vi "Generate Self-Signed Certificates.vi"() -> ()   [LabVIEW 2013]
uses:
  certificate -- cluster.ctl
  certificate signature request (CA) -- cluster.ctl
  encryption key -- cluster.ctl
  initca -- cluster.ctl
  certificate signature request (Server) -- cluster.ctl
  <vilib>/Platform/browser.llb/Open URL in Default Browser (path).vi
  <userlib>/_OpenG.lib/file/file.llb/Build Path - Traditional__ogtk.vi
  <userlib>/_OpenG.lib/file/file.llb/File Exists - Scalar__ogtk.vi
  <userlib>/_OpenG.lib/file/file.llb/Convert File Extension (String)__ogtk.vi
panel:
  out "Selected Certificate":string
  in  "Certificates and Keys":i32(listbox)
  in  "Open Explorer":bool
  in  "Servers":cluster{"hosts":string[], "name":string}[](array[cluster])
  in  "Root Private Key":path
  in  "Root Certificate":path
  in  "Generate Server Certificates":bool
  in  "Generate Root Certificate":bool
  in  "Common Name":string="lvtls-ca.example"
  in  "Hosts":string[](array[string])=["lvtls-ca.example", "www.lvtls-ca.example"]
  # "1- ROOT (CERTIFICATE AUTHORITY)\nIf you have a root certificate and private key, import it to generate server certificate files.\nIf you don't have a root certificate, fill in the fields below and generate one."
  # "3- SERVERS\nList each server you want to create certificates for."
  # "2- GENERATE ROOT CERTIFICATE\nIf you don't have a root certificate, fill in the fields below and generate one."
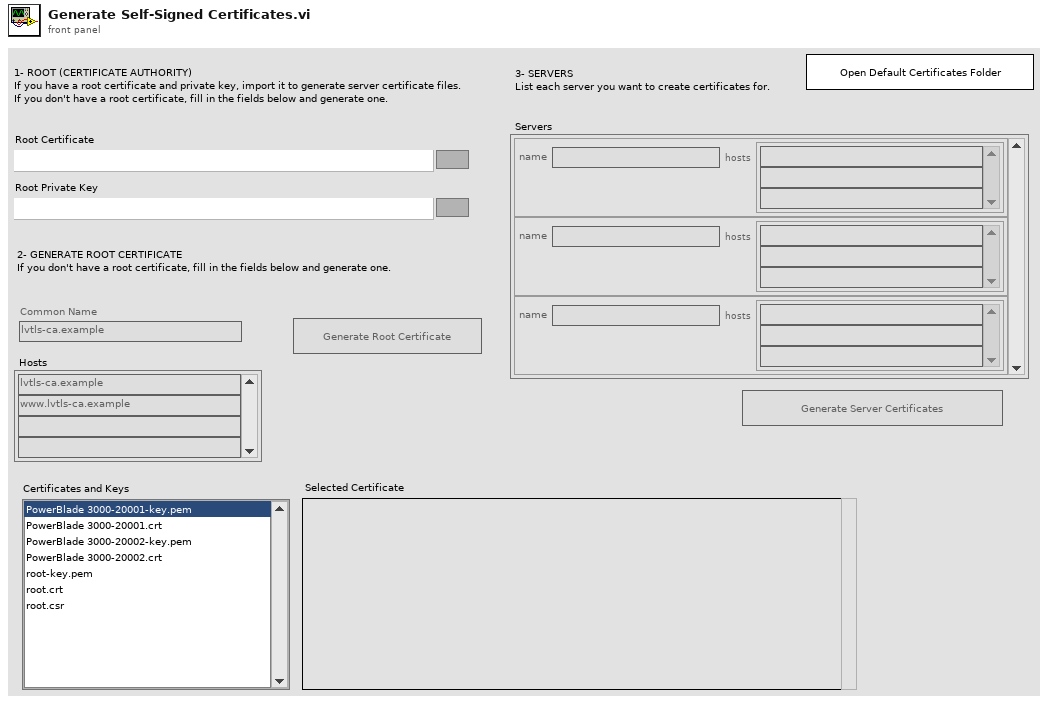
[diagram p1: front panel]
types:
  T1 = enum32{"Invalid", "Standard", "Closed", "Hidden", "Minimized", "Maximized"}
  T2 = enum32{"invalid app kind", "Development System", "Run Time System", "Student Edition", "Embedded LabVIEW", "Evaluation", "Custom"}
  T3 = enum16{"open", "replace", "create", "open or create", "replace or create", "replace or create with confirmation"}
  T4 = typedef "certificate signature request (CA) -- cluster.ctl" = cluster{"CN":string, "hosts":string[], "key":T5, "ca":T6}
  T5 = typedef "encryption key -- cluster.ctl" = cluster{"algo":string, "size":u32}
  T6 = typedef "initca -- cluster.ctl" = cluster{"pathlen":u8, "expiry":string}
  T7 = typedef "certificate signature request (Server) -- cluster.ctl" = cluster{"CN":string, "hosts":string[], "key":T5}
  T8 = typedef "certificate -- cluster.ctl" = cluster{"cert":string, "csr":string, "key":string}
  T9 = cluster{"Core":cluster{"Current VI Reference":refnum<vi>, "Close Panel on Exit?":bool}, "CA":T8, "Server":T8, "cfssl path":path, "temp folder":path, "Certificates Folder":path, "Root name":string, "Root Certificate":path, "Root Private Key":path, "Active CN":string, "Active Hosts":string[], "next":i32, "Processing Queue":cluster{"hosts":string[], "name":string}[]}
  T10 = cluster{"Current VI Reference":refnum<vi>, "Close Panel on Exit?":bool}
  T11 = enum8{"Enabled", "Disabled", "Disabled and Grayed Out"}
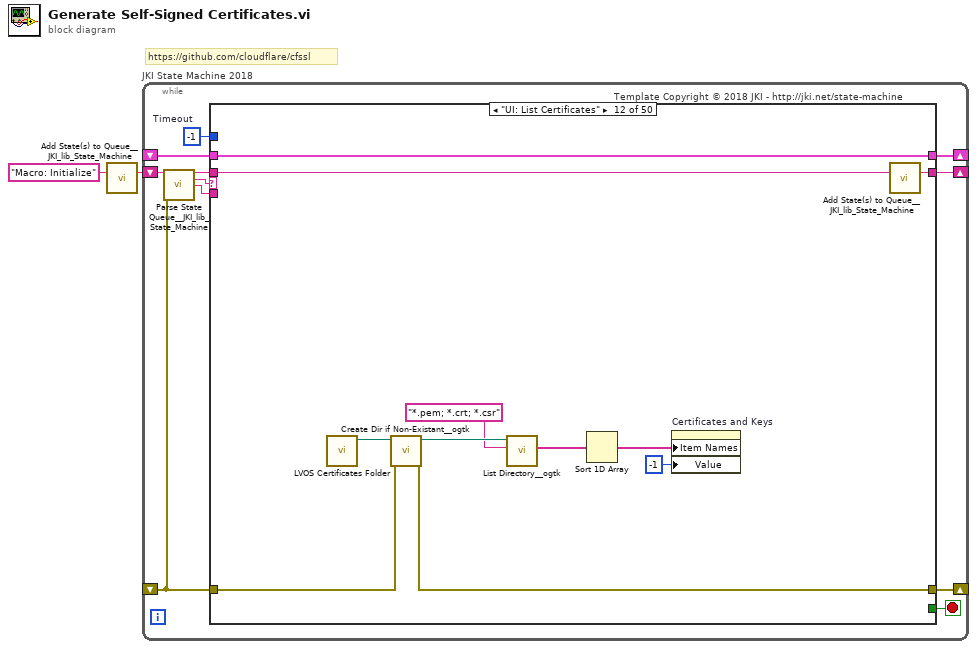
[diagram p0: block diagram]
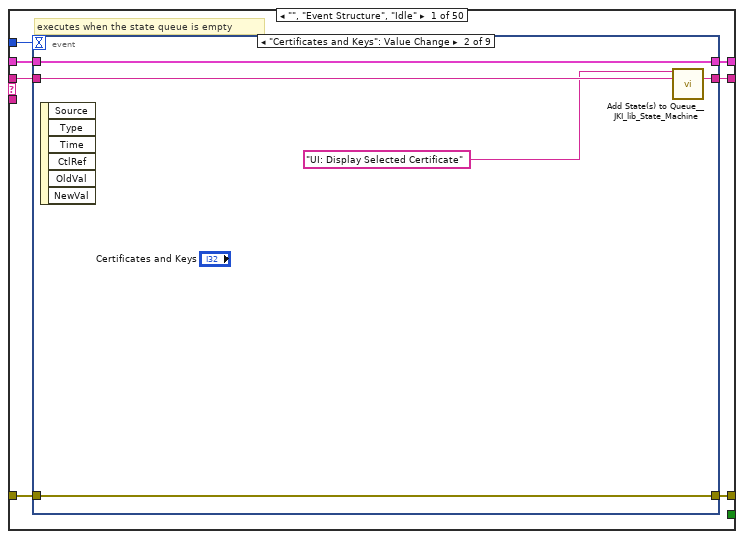
[diagram p2: hidden frame]
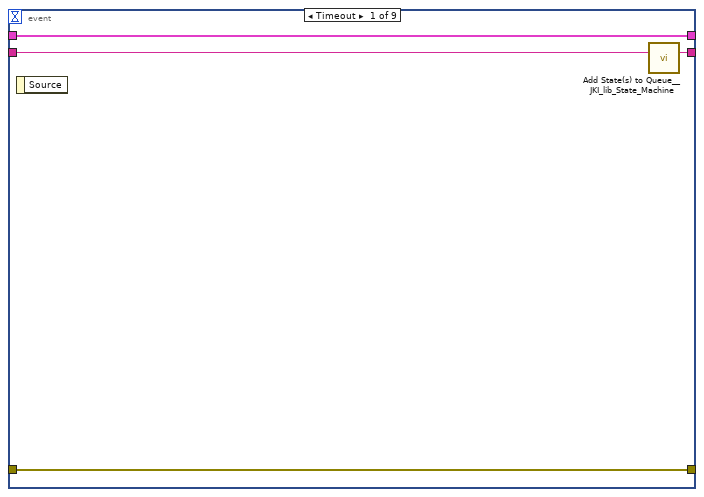
[diagram p3: hidden frame]
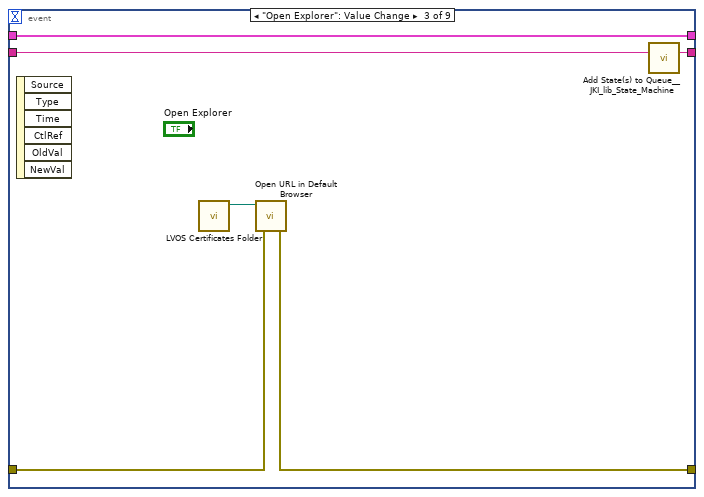
[diagram p4: hidden frame]
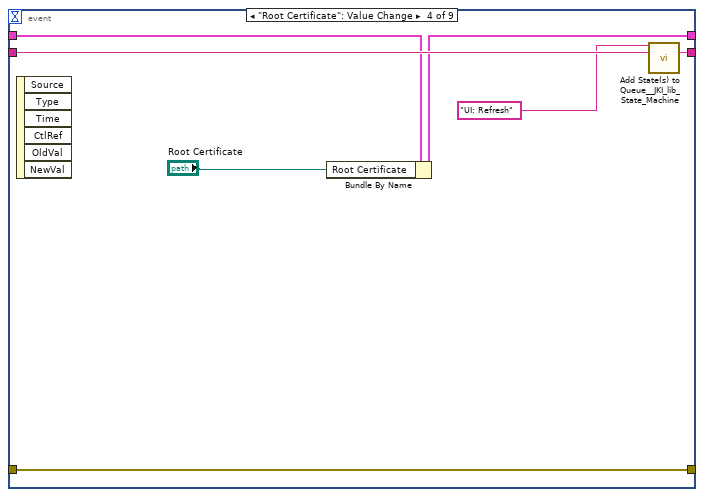
[diagram p5: hidden frame]
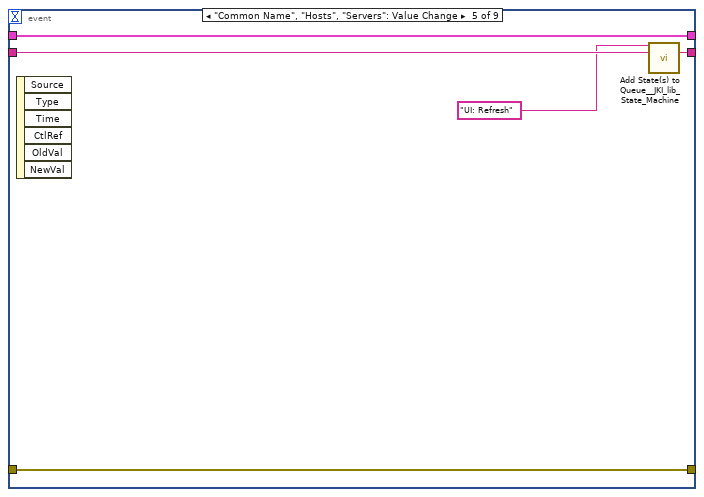
[diagram p6: hidden frame]
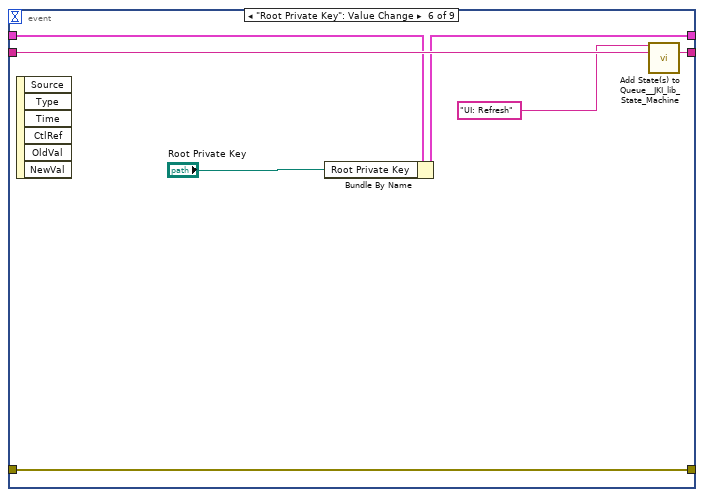
[diagram p7: hidden frame]
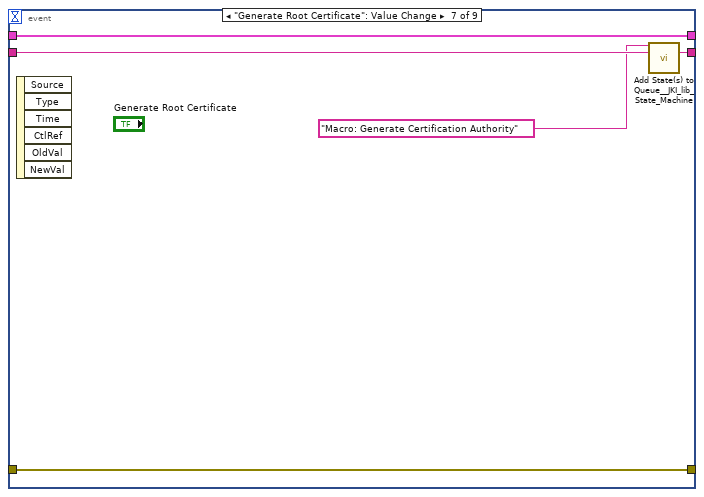
[diagram p8: hidden frame]
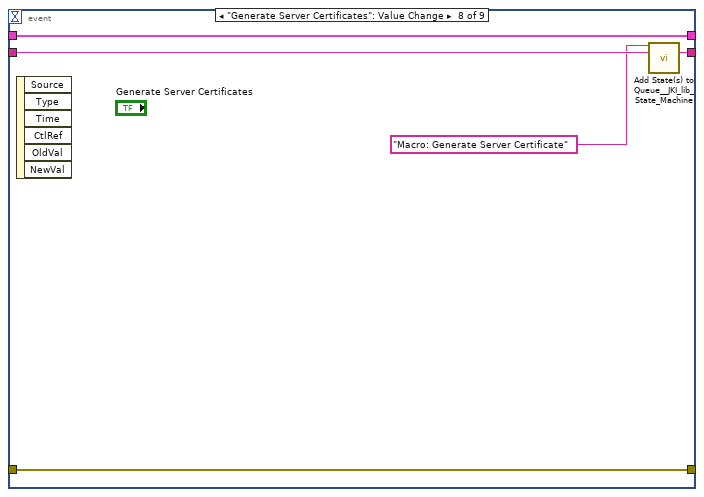
[diagram p9: hidden frame]
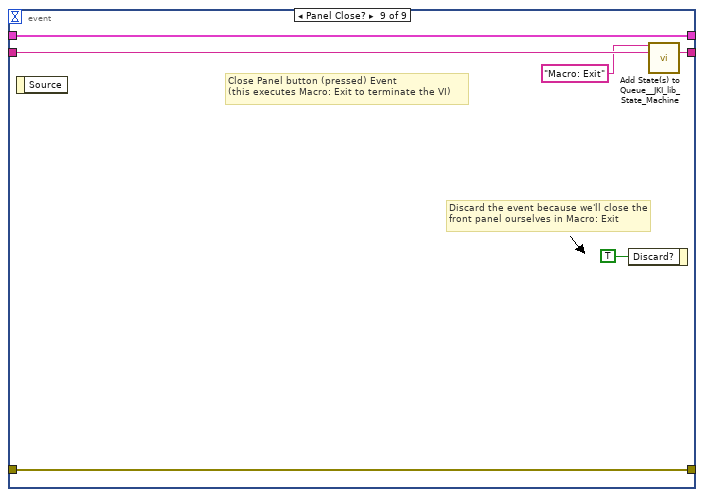
[diagram p10: hidden frame]
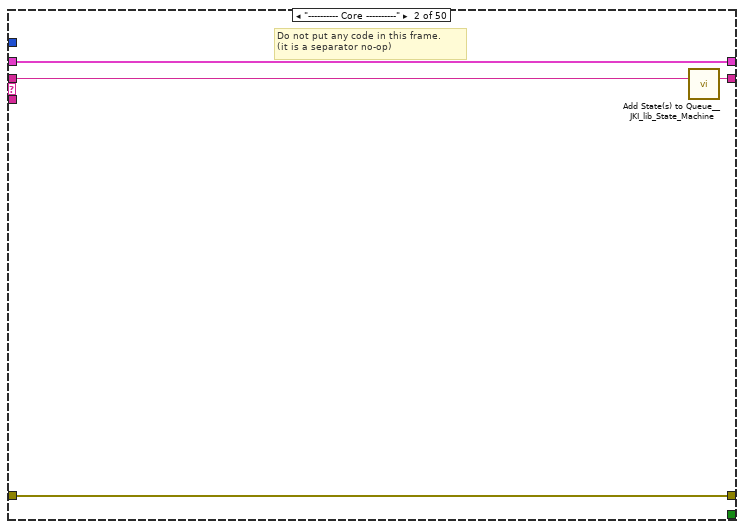
[diagram p11: hidden frame]
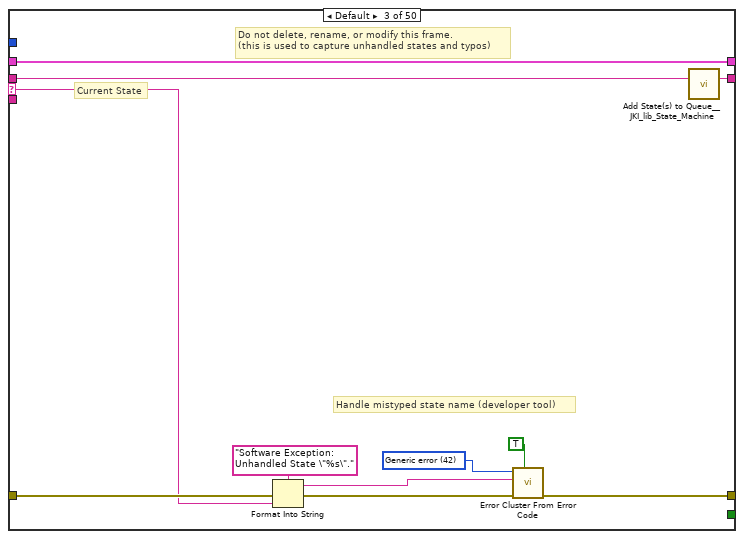
[diagram p12: hidden frame]
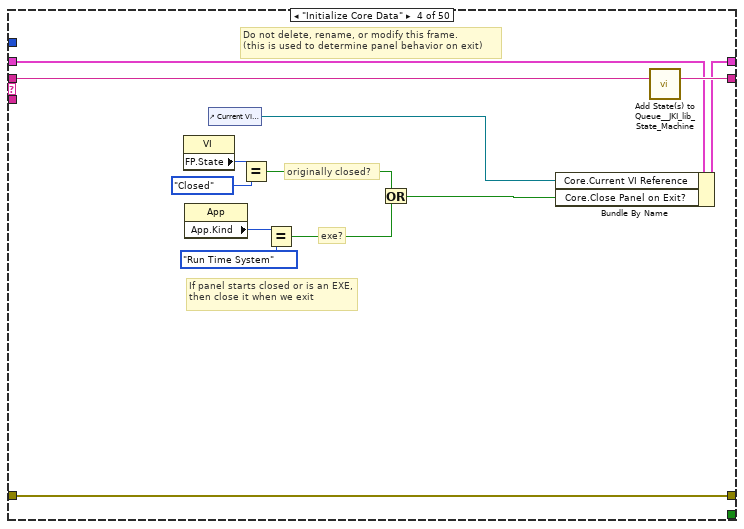
[diagram p13: hidden frame]
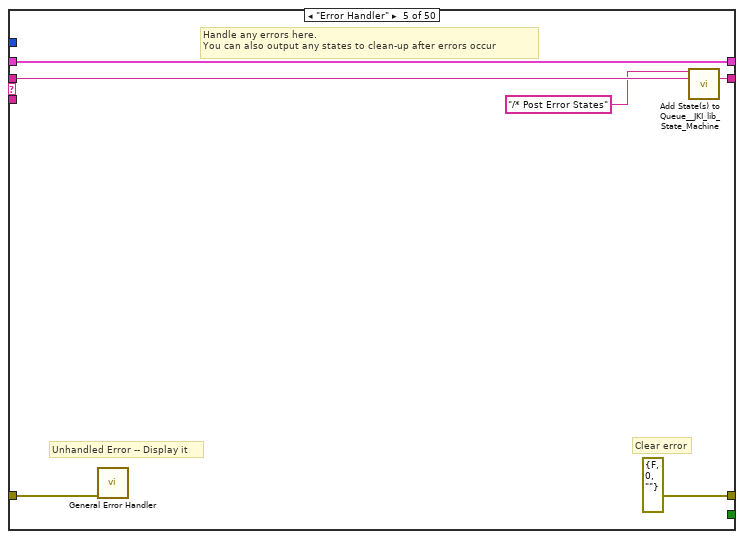
[diagram p14: hidden frame]
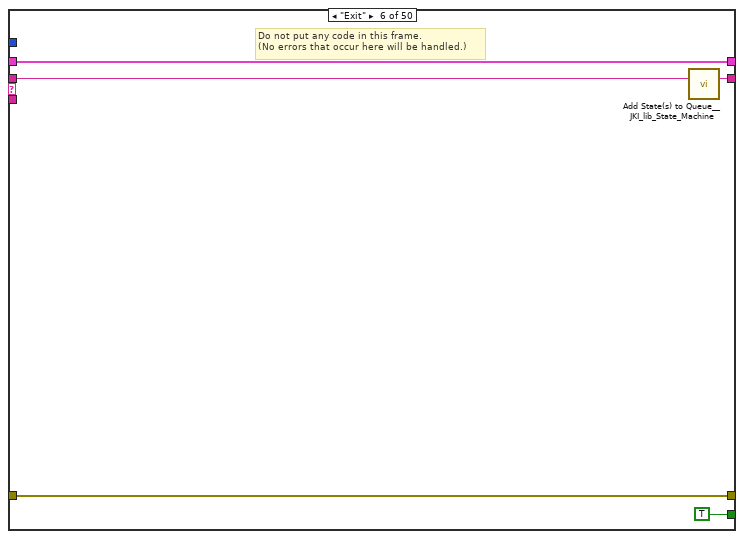
[diagram p15: hidden frame]
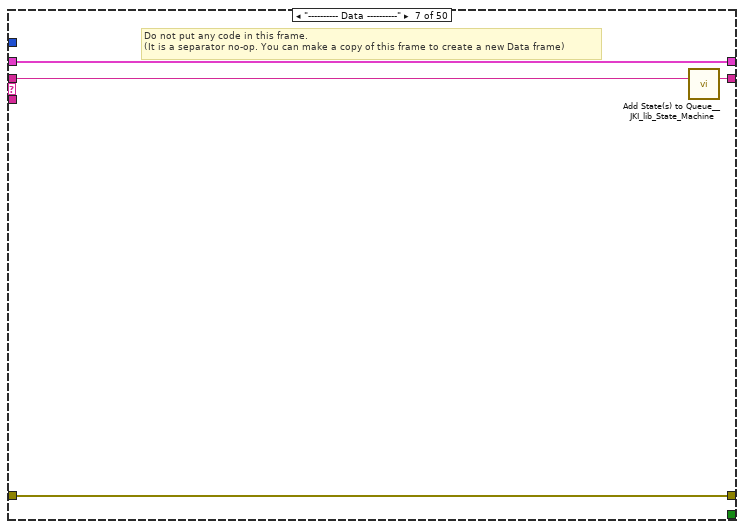
[diagram p16: hidden frame]
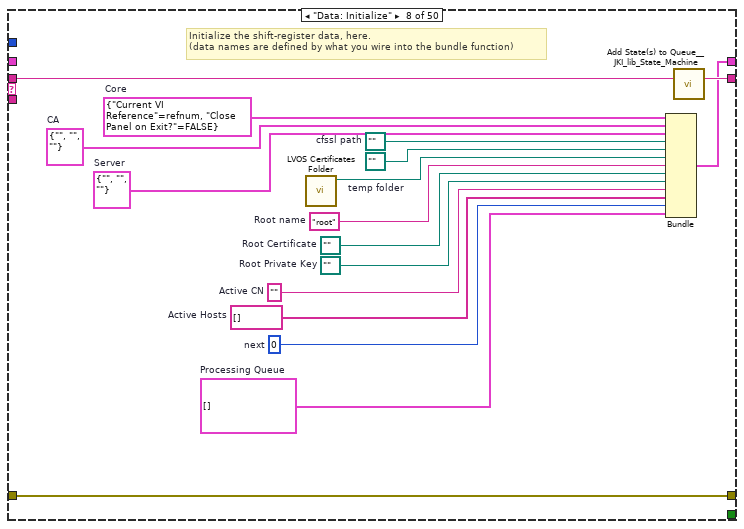
[diagram p17: hidden frame]
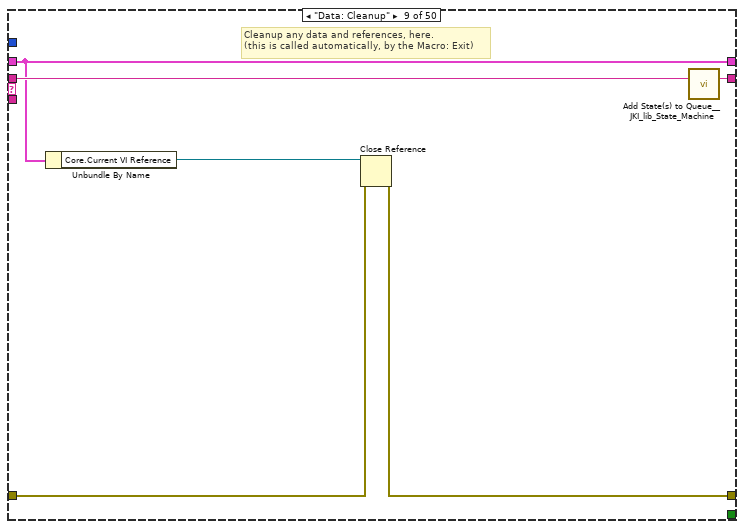
[diagram p18: hidden frame]
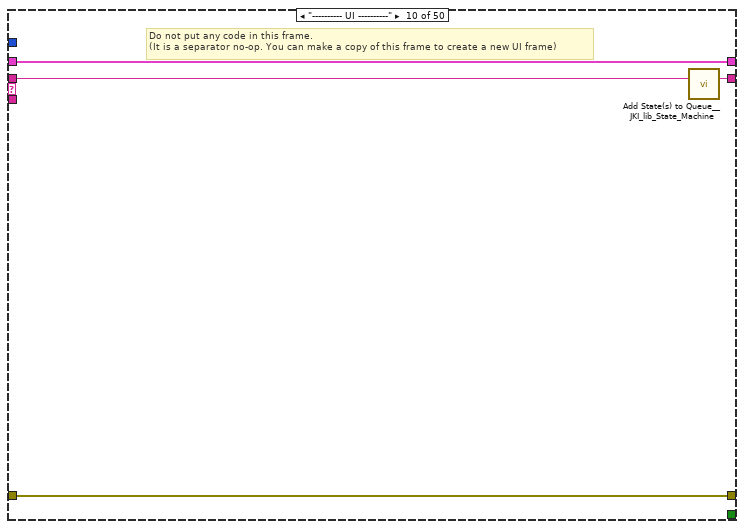
[diagram p19: hidden frame]
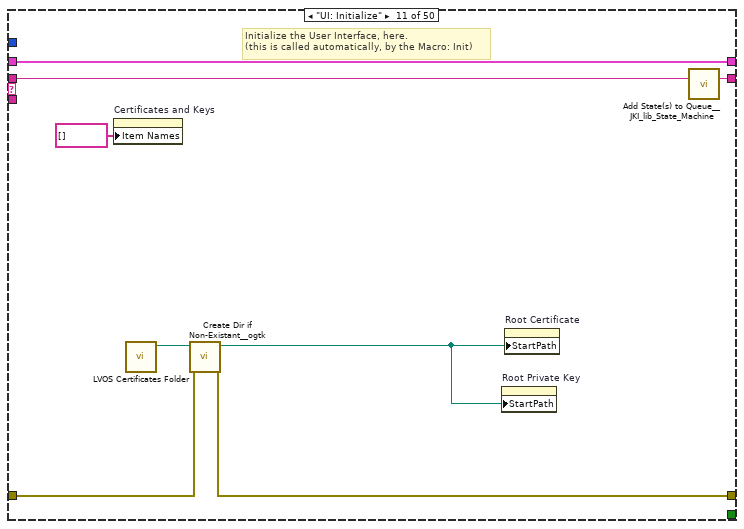
[diagram p20: hidden frame]
diagram:
  # "https://github.com/cloudflare/cfssl"
  n1 = call <vilib>:"Add State(s) to Queue__JKI_lib_State_Machine.vi"("State(s) in (\"\")"="Macro: Initialize") -> ("States Out"=w2:string)  [unwired: 14 in]
  n2 = while "JKI State Machine 2018" {
    shift-right: [w6] -> _
    shift-left: _ -> [w5]
    shift-right: [w9] -> _
    shift-left: _ -> [w3]
    shift-right: [w8] -> _
    shift-left: w2 -> [w10]
    stop <- w7 stop-if-true
    w4 = -1  # Timeout
    # "Template Copyright © 2018 JKI - http://jki.net/state-machine"
    n3 = call <vilib>:"Parse State Queue__JKI_lib_State_Machine.vi"("State Queue"=w10, "Error In (no error)"=w3) -> ("Remaining States"=w12:string, "Current State"=w13:string, "Arguments"=w11:string)  [unwired: 11 in]
    n4 = case shown="\"UI: List Certificates\"" w13 {
      selector: w13 -> [_ _ w75 _ _ _ _ _ _ _ _ _ _ _ _ _ _ _ _ _ _ _ _ _ _ _ _ _ _ _ _ _ _ _ _ _ _ _ _ _ _ _ _ _ _ _ _ _ _ _]
      tunnel: w12 -> [w20 w74 w79 w98 w104 w109 w113 w130 w136 w140 w148 w159 w167 w217 w221 w225 w230 w236 w247 w316 w321 w326 w334 w339 w348 w353 w364 w368 w376 w385 w395 w422 w437 w452 w475 w496 w513 w523 w537 w568 w591 w617 w640 w672 w689 w706 w723 w740 w757 w774]
      tunnel: w11 -> [_ _ _ _ _ _ _ _ _ _ _ _ _ _ _ _ _ w231 w241 _ _ _ _ _ _ _ _ _ _ _ _ _ _ _ _ _ _ _ _ _ _ _ _ _ _ _ _ _ _ _]
      tunnel: w5 -> [w18 w71 w77 w91 w101 w107 w110 _ w131 w137 w146 w157 w165 w206 w218 w222 w227 w234 w243 w313 w318 w323 w330 w336 w345 w350 w361 w365 w373 w383 w393 w418 w426 w442 w473 w494 w506 w518 w535 w538 w584 w613 w630 w655 w681 w698 w715 w732 w749 w766]
      tunnel: [w17 w72 w81 w95 errorcluster {"status"=FALSE, "code"=0, "source"=""} ("error out") w106 w111 w127 w132 w138 w142 w154 w162 w215 w219 w223 w228 w232 w244 w314 w319 w324 w332 w337 w346 w351 w362 w366 w374 w378 w389 w420 w423 w439 w453 w482 w499 w514 w526 w541 w586 w614 w619 w656 w676 w693 w710 w727 w744 w761] -> w9
      tunnel: w3 -> [w16 w72 w80 w95 w100 w106 w111 w127 w133 w138 w143 w155 w162 w215 w219 w223 w228 w233 w245 w314 w319 w324 w332 w337 w346 w351 w362 w366 w374 w379 w388 w420 w424 w440 w454 w483 w500 w514 w524 w545 w587 w615 w622 w659 w678 w695 w712 w729 w746 w763]
      tunnel: [w19 w73 w78 w97 w103 w108 w112 w129 w135 w139 w147 w158 w166 w216 w220 w224 w229 w235 w246 w315 w320 w325 w333 w338 w347 w352 w363 w367 w375 w384 w394 w421 w436 w451 w474 w495 w512 w522 w536 w567 w590 w616 w639 w671 w688 w705 w722 w739 w756 w773] -> w8
      tunnel: [_ _ _ _ _ TRUE _ _ _ _ _ _ _ _ _ _ _ _ _ _ _ _ _ _ _ _ _ _ _ _ _ _ _ _ _ _ _ _ _ _ _ _ _ _ _ _ _ _ _ _] -> w7
      tunnel: [w15 w71 w77 w96 w101 w107 w110 w128 w131 w137 w146 w157 w165 w206 w218 w222 w227 w234 w243 w313 w318 w323 w329 w336 w345 w350 w361 w365 w372 w382 w393 w419 w427 w443 w473 w494 w506 w521 w535 w538 w583 w612 w630 w655 w681 w698 w715 w732 w749 w766] -> w6
      tunnel: w4 -> [w14 _ _ _ _ _ _ _ _ _ _ _ _ _ _ _ _ _ _ _ _ _ _ _ _ _ _ _ _ _ _ _ _ _ _ _ _ _ _ _ _ _ _ _ _ _ _ _ _ _]
      frame "", "Event Structure", "Idle" {
        # "executes when the state queue is empty"
        n5 = event shown="[1] \"Certificates and Keys\": Value Change" {
          selector: _ -> [_ _ _ _ _ _ _ _ _]
          dyn-events: _ -> [_ _ _ _ _ _ _ _ _]
          timeout: w14 -> [_ _ _ _ _ _ _ _ _]
          tunnel: w20 -> [w24 w29 w35 w42 w47 w54 w59 w64 w70]
          tunnel: [w23 w28 w34 w41 w46 w53 w58 w63 w69] -> w19
          tunnel: w18 -> [w21 w26 w33 w39 w43 w51 w56 w61 w67]
          tunnel: [w22 w27 w30 w40 w45 w52 w57 w62 w68] -> w17
          tunnel: w16 -> [w22 w27 w31 w40 w45 w52 w57 w62 w68]
          tunnel: [w21 w26 w33 w38 w43 w50 w56 w61 w67] -> w15
          event Timeout {
            n6 = event-data() -> ()  [unwired: 1 in, 1 out]
            n7 = call <vilib>:"Add State(s) to Queue__JKI_lib_State_Machine.vi"("State(s) in (\"\")"=w24) -> ("States Out"=w23:string)  [unwired: 14 in]
          }
          event "Certificates and Keys": Value Change {
            n8 = event-data() -> ()  [unwired: 1 in, 6 out]
            n9 = call <vilib>:"Add State(s) to Queue__JKI_lib_State_Machine.vi"("State(s) in Front (\"\")"="UI: Display Selected Certificate", "State(s) in (\"\")"=w29) -> ("States Out"=w28:string)  [unwired: 13 in]
          }
          event "Open Explorer": Value Change {
            n10 = event-data() -> ()  [unwired: 1 in, 6 out]
            n11 = call "LVOS Certificates Folder.vi"() -> ("Certificates Folder"=w32:path)  [unwired: 11 in]
            n12 = call-poly <vilib>:"Open URL in Default Browser.vi"("error in (no error)"=w31, "path"=w32) -> ("error out"=w30:errorcluster)  [unwired: 4 in, 1 out]
            n13 = call <vilib>:"Add State(s) to Queue__JKI_lib_State_Machine.vi"("State(s) in (\"\")"=w35) -> ("States Out"=w34:string)  [unwired: 14 in]
          }
          event "Root Certificate": Value Change {
            n14 = event-data() -> ()  [unwired: 1 in, 6 out]
            n15 = Bundle By Name(cluster=w39, "Root Certificate"="Root Certificate") -> (w38:T9)
            n16 = call <vilib>:"Add State(s) to Queue__JKI_lib_State_Machine.vi"("State(s) in Front (\"\")"="UI: Refresh", "State(s) in (\"\")"=w42) -> ("States Out"=w41:string)  [unwired: 13 in]
          }
          event "Common Name", "Hosts", "Servers": Value Change {
            n17 = event-data() -> ()  [unwired: 1 in, 6 out]
            n18 = call <vilib>:"Add State(s) to Queue__JKI_lib_State_Machine.vi"("State(s) in Front (\"\")"="UI: Refresh", "State(s) in (\"\")"=w47) -> ("States Out"=w46:string)  [unwired: 13 in]
          }
          event "Root Private Key": Value Change {
            n19 = event-data() -> ()  [unwired: 1 in, 6 out]
            n20 = Bundle By Name(cluster=w51, "Root Private Key"="Root Private Key") -> (w50:T9)
            n21 = call <vilib>:"Add State(s) to Queue__JKI_lib_State_Machine.vi"("State(s) in Front (\"\")"="UI: Refresh", "State(s) in (\"\")"=w54) -> ("States Out"=w53:string)  [unwired: 13 in]
          }
          event "Generate Root Certificate": Value Change {
            n22 = event-data() -> ()  [unwired: 1 in, 6 out]
            n23 = call <vilib>:"Add State(s) to Queue__JKI_lib_State_Machine.vi"("State(s) in Front (\"\")"="Macro: Generate Certification Authority", "State(s) in (\"\")"=w59) -> ("States Out"=w58:string)  [unwired: 13 in]
          }
          event "Generate Server Certificates": Value Change {
            n24 = event-data() -> ()  [unwired: 1 in, 6 out]
            n25 = call <vilib>:"Add State(s) to Queue__JKI_lib_State_Machine.vi"("State(s) in Front (\"\")"="Macro: Generate Server Certificate", "State(s) in (\"\")"=w64) -> ("States Out"=w63:string)  [unwired: 13 in]
          }
          event Panel Close? {
            # "Discard the event because we'll close the front panel ourselves in Macro: Exit"
            # "Close Panel button (pressed) Event\n(this executes Macro: Exit to terminate the VI)"
            n26 = event-data() -> ()  [unwired: 1 in, 1 out]
            n27 = event-data("Discard?"=TRUE) -> ()  [unwired: 1 in, 1 out]
            n28 = call <vilib>:"Add State(s) to Queue__JKI_lib_State_Machine.vi"("State(s) in Front (\"\")"="Macro: Exit", "State(s) in (\"\")"=w70) -> ("States Out"=w69:string)  [unwired: 13 in]
          }
        }
      }
      frame "---------- Core ----------" {
        # "Do not put any code in this frame.\n(it is a separator no-op)"
        n29 = call <vilib>:"Add State(s) to Queue__JKI_lib_State_Machine.vi"("State(s) in (\"\")"=w74) -> ("States Out"=w73:string)  [unwired: 14 in]
      }
      frame Default {
        w84 = 42 items=["No error", "Argument error", "Memory is full", "Out of zone", "End of file", "File already open", "Generic file I/O error", "File not found", "File permission error", "Disk is full", "Duplicate path", "Too many files open", "System feature not enabled", "Resource file not found", "Cannot add resource", "Resource not found", "Image not found", "Image memory error", "Pen does not exist", "Config type invalid", "Config token not found", "Config parse error", "Config memory error", "Bad external code format", "Bad external code offset", "External code not present", "Null window", "Destroy window error", "Null menu", "Print aborted", "Bad print record", "Print driver error", "Windows error during printing", "Memory error during printing", "Print dialog error", "Generic print error", "Invalid device refnum", "Device not found", "Device parameter error", "Device unit error", "Cannot open device", "Device call aborted", "Generic error", "Cancelled by user", "Object ID too low", "Object ID too high", "Object not in heap", "Unknown heap", "Unknown object (invalid DefProc)", "Unknown object (DefProc not in table)", "Message out of range", "Invalid (null) method", "Unknown message", "Manager call not supported", "Bad address", "Network operation in progress", "Network operation timed out", "Connection is busy", "Network attribute not supported", "Network error", "Address in use", "System out of memory", "Connection aborted", "Connection refused", "Not connected", "Already connected", "Connection closed", "Initialization error (interapplication manager)", "Bad occurrence", "Wait on unbound occurrence handler", "Occurrence queue overflow", "Datalog type conflict", "Unused", "Unrecognized type (interapplication manager)", "Memory corrupt", "Failed to make temporary DLL", "Old CIN version", "Drag socket not found", "Failed to load drop-object", "Failed to register OLE object", "Failed to release OLE object", "Format specifier type mismatch", "Unknown format specifier", "Too few format specifiers", "Too many format specifiers", "Scan failed", "Newer CIN version", "Error converting to variant", "Runtime menu error", "Password tampered", "Variant attribute not found", "Incompatible variant data type", "Event data is not available", "Event Store is not present", "Occurrence is not found", "Event Queue is not created", "Event info is not available", "Refnum passed is NULL", "Error retrieving Class GUID", "Error retrieving CoClass GUID", "Error retrieving TypeLib GUID.", "Bad built application magic bytes.", "Specific driver is different from the specific driver associated with the Logical Name.", "There is no session opened to the class driver.", "Max Error", "MAX - Error with config objects", "MAX - Error loading configuration", "MAX - Group not supported"]
        # "Current State"
        # "Do not delete, rename, or modify this frame.\n(this is used to capture unhandled states and typos)"
        # "Handle mistyped state name (developer tool)"
        n30 = Format Into String(format string="Software Exception: Unhandled State \"%s\"." ("message"), error in=w80, w75) -> (resulting string=w83:string, error out=w82:errorcluster)  [unwired: 1 in]
        n31 = call <vilib>:"Error Cluster From Error Code.vi"("show call chain? (False)"=TRUE, "error in (no error)"=w82, "error message (\"\")"=w83, "error code (0)"=w84) -> ("error out"=w81:errorcluster)  [unwired: 5 in]
        n32 = call <vilib>:"Add State(s) to Queue__JKI_lib_State_Machine.vi"("State(s) in (\"\")"=w79) -> ("States Out"=w78:string)  [unwired: 14 in]
      }
      frame "Initialize Core Data" {
        # "Do not delete, rename, or modify this frame.\n(this is used to determine panel behavior on exit)"
        # "originally closed?"
        # "exe?"
        # "If panel starts closed or is an EXE, then close it when we exit"
        n33 = property class="VI"() -> ("FP.State"=w88:T1)  [unwired: 2 in, 2 out]
        n34 = property class="App"() -> ("App.Kind"=w94:T2)  [unwired: 2 in, 2 out]
        n35 = control-ref of="Current VI Reference"() -> (w89:refnum<vi>)
        n36 = Equal?(x=w88, y=T1."Closed" ("Front Panel Window:State")) -> (x = y?=w86:bool)
        n37 = Equal?(x=w94, y=T2."Run Time System" ("Application:Kind")) -> (x = y?=w92:bool)
        n38 = Or(x=w86, y=w92) -> (x .or. y?=w90:bool)
        n39 = Bundle By Name(cluster=w91, "Core.Current VI Reference"=w89, "Core.Close Panel on Exit?"=w90) -> (w96:T9)
        n40 = call <vilib>:"Add State(s) to Queue__JKI_lib_State_Machine.vi"("State(s) in (\"\")"=w98) -> ("States Out"=w97:string)  [unwired: 14 in]
      }
      frame "Error Handler" {
        # "Unhandled Error -- Display it"
        # "Handle any errors here.\nYou can also output any states to clean-up after errors occur"
        # "Clear error"
        n41 = call <vilib>:"General Error Handler.vi"("error in (no error)"=w100) -> ()  [unwired: 10 in, 5 out]
        n42 = call <vilib>:"Add State(s) to Queue__JKI_lib_State_Machine.vi"("State(s) in Front (\"\")"="/* Post Error States", "State(s) in (\"\")"=w104) -> ("States Out"=w103:string)  [unwired: 13 in]
      }
      frame "Exit" {
        # "Do not put any code in this frame.\n(No errors that occur here will be handled.)"
        n43 = call <vilib>:"Add State(s) to Queue__JKI_lib_State_Machine.vi"("State(s) in (\"\")"=w109) -> ("States Out"=w108:string)  [unwired: 14 in]
      }
      frame "---------- Data ----------" {
        # "Do not put any code in this frame.\n(It is a separator no-op. You can make a copy of this frame to create a new Data frame)"
        n44 = call <vilib>:"Add State(s) to Queue__JKI_lib_State_Machine.vi"("State(s) in (\"\")"=w113) -> ("States Out"=w112:string)  [unwired: 14 in]
      }
      frame "Data: Initialize" {
        w114 = cluster{"hosts":string[], "name":string}[] []  # Processing Queue
        w115 = 0  # next
        w117 = string[] []  # Active Hosts
        w118 = ""  # Active CN
        w119 = path ""  # Root Private Key
        w120 = path ""  # Root Certificate
        w121 = "root"  # Root name
        w122 = path ""  # temp folder
        w123 = path ""  # cfssl path
        w124 = T8 {"cert"="", "csr"="", "key"=""}  # Server
        w125 = T8 {"cert"="", "csr"="", "key"=""}  # CA
        w126 = T10 {"Current VI Reference"=refnum, "Close Panel on Exit?"=FALSE}  # Core
        # "Initialize the shift-register data, here.\n(data names are defined by what you wire into the bundle function)"
        n45 = call "LVOS Certificates Folder.vi"() -> ("Certificates Folder"=w116:path)  [unwired: 11 in]
        n46 = Bundle("Core"=w126, "CA"=w125, "Server"=w124, "cfssl path"=w123, "temp folder"=w122, "Certificates Folder"=w116, "Root name"=w121, "Root Certificate"=w120, "Root Private Key"=w119, "Active CN"=w118, "Active Hosts"=w117, "next"=w115, "Processing Queue"=w114) -> (w128:T9)  [unwired: 1 in]
        n47 = call <vilib>:"Add State(s) to Queue__JKI_lib_State_Machine.vi"("State(s) in (\"\")"=w130) -> ("States Out"=w129:string)  [unwired: 14 in]
      }
      frame "Data: Cleanup" {
        # "Cleanup any data and references, here.\n(this is called automatically, by the Macro: Exit)"
        n48 = Unbundle By Name(w131) -> ("Core.Current VI Reference"=w134:refnum<vi>)
        n49 = Close Reference(reference=w134, error in (no error)=w133) -> (error out=w132:errorcluster)
        n50 = call <vilib>:"Add State(s) to Queue__JKI_lib_State_Machine.vi"("State(s) in (\"\")"=w136) -> ("States Out"=w135:string)  [unwired: 14 in]
      }
      frame "---------- UI ----------" {
        # "Do not put any code in this frame.\n(It is a separator no-op. You can make a copy of this frame to create a new UI frame)"
        n51 = call <vilib>:"Add State(s) to Queue__JKI_lib_State_Machine.vi"("State(s) in (\"\")"=w140) -> ("States Out"=w139:string)  [unwired: 14 in]
      }
      frame "UI: Initialize" {
        # "Initialize the User Interface, here.\n(this is called automatically, by the Macro: Init)"
        n52 = property on="Certificates and Keys" class="LstBox (strict)"("Item Names"=string[] []) -> ()  [unwired: 2 in, 2 out]
        n53 = call "LVOS Certificates Folder.vi"() -> ("Certificates Folder"=w145:path)  [unwired: 11 in]
        n54 = call <userlib>:"Create Dir if Non-Existant__ogtk.vi"("error in (no error)"=w143, "Directory Path"=w145) -> ("error out"=w142:errorcluster, "dup Directory Path"=w144:path)  [unwired: 7 in, 1 out]
        n55 = property on="Root Private Key" class="Path"("StartPath"=w144) -> ()  [unwired: 2 in, 2 out]
        n56 = property on="Root Certificate" class="Path"("StartPath"=w144) -> ()  [unwired: 2 in, 2 out]
        n57 = call <vilib>:"Add State(s) to Queue__JKI_lib_State_Machine.vi"("State(s) in (\"\")"=w148) -> ("States Out"=w147:string)  [unwired: 14 in]
      }
      frame "UI: List Certificates" {
        n58 = call "LVOS Certificates Folder.vi"() -> ("Certificates Folder"=w156:path)  [unwired: 11 in]
        n59 = call <userlib>:"Create Dir if Non-Existant__ogtk.vi"("error in (no error)"=w155, "Directory Path"=w156) -> ("error out"=w154:errorcluster, "dup Directory Path"=w153:path)  [unwired: 7 in, 1 out]
        n60 = call <userlib>:"List Directory__ogtk.vi"("pattern"="*.pem; *.crt; *.csr", "directory path"=w153) -> ("file names"=w151:string[])  [unwired: 2 in, 3 out]
        n61 = Sort 1D Array(array=w151) -> (sorted array=w150:string[])
        n62 = property on="Certificates and Keys" class="LstBox (strict)"("Item Names"=w150, "Value"=-1 ("Trusted Certificates")) -> ()  [unwired: 2 in, 2 out]
        n63 = call <vilib>:"Add State(s) to Queue__JKI_lib_State_Machine.vi"("State(s) in (\"\")"=w159) -> ("States Out"=w158:string)  [unwired: 14 in]
      }
      frame "UI: Display Selected Certificate" {
        n64 = property on="Certificates and Keys" class="LstBox (strict)"() -> ("Item Names"=w164:string[], "Value"=w163:i32)  [unwired: 2 in, 2 out]
        n65 = Index Array(array=w164, index=w163) -> (element=w161:string)
        n66 = case shown="Default" w161 {
          selector: w161 -> [w174 _]
          tunnel: [w168 _] -> w160
          frame Default {
            n67 = call "LVOS Certificates Folder.vi"() -> ("Certificates Folder"=w175:path)  [unwired: 11 in]
            n68 = call-poly <userlib>:"Build Path__ogtk.vi"("name or relative path"=w174, "base path"=w175) -> ("appended path"=w170:path)
            n69 = call-poly <userlib>:"File Exists__ogtk.vi"("file path"=w170) -> ("is directory"=w173:bool, "exists"=w172:bool)  [unwired: 6 in]
            n70 = Empty String/Path?(string/path=w170) -> (empty?=w171:bool)
            n71 = Compound Arithmetic op=AND(invert w173, w172, invert w171) -> (w169:bool)
            n72 = case shown="True" w169 {
              tunnel: w170 -> [_ w177]
              tunnel: [_ w176] -> w168
              frame False {
              }
              frame True {
                n73 = Open/Create/Replace File(file path (use dialog)=w177, operation (0:open)=T3."open", access (0:read/write)=enum16{"read/write", "read-only", "write-only"}."read-only") -> (refnum out=w182:refnum<file>, error out=w183:errorcluster)  [unwired: 3 in, 1 out]
                n74 = Read from Text File(file (use dialog)=w182, error in=w183) -> (refnum out=w180:refnum<file>, text=w176:string, error out=w181:errorcluster)  [unwired: 2 in, 1 out]
                n75 = Close File(refnum=w180, error in=w181) -> ()  [unwired: 2 out]
              }
            }
          }
          frame "\u0000" {
          }
        }
        "Selected Certificate" <- w160
        n76 = call <vilib>:"Add State(s) to Queue__JKI_lib_State_Machine.vi"("State(s) in (\"\")"=w167) -> ("States Out"=w166:string)  [unwired: 14 in]
      }
      frame "UI: Refresh" {
        w189 = T11."Disabled and Grayed Out" ("Disabled")
        w188 = T11."Enabled" ("Disabled")
        n77 = Unbundle By Name(w206) -> ("Certificates Folder"=w212:path)
        n78 = Unbundle By Name(w206) -> ("Root Certificate"=w185:path, "Root Private Key"=w184:path)
        n79 = local read "Common Name"() -> (w195:string)
        n80 = local read "Servers"() -> (w209:cluster{"hosts":string[], "name":string}[])
        n81 = local read "Hosts"() -> (w194:string[])
        n82 = local write "Root Private Key"(w184) -> ()
        n83 = call-poly <userlib>:"File Exists__ogtk.vi"("file path"=w212) -> ("is directory"=w210:bool, "exists"=w211:bool)  [unwired: 6 in]
        n84 = Empty String/Path?(string/path=w212) -> (empty?=w213:bool)
        n85 = Empty Array?(array=w209) -> (empty?=w214:bool)
        n86 = Empty String/Path?(string/path=w195) -> (empty?=w191:bool)
        n87 = local write "Root Certificate"(w185) -> ()
        n88 = call-poly <userlib>:"File Exists__ogtk.vi"("file path"=w185) -> ("is directory"=w205:bool, "exists"=w204:bool)  [unwired: 6 in]
        n89 = call-poly <userlib>:"File Exists__ogtk.vi"("file path"=w184) -> ("is directory"=w200:bool, "exists"=w201:bool)  [unwired: 6 in]
        n90 = Empty String/Path?(string/path=w185) -> (empty?=w203:bool)
        n91 = Empty String/Path?(string/path=w184) -> (empty?=w202:bool)
        n92 = Empty Array?(array=w194) -> (empty?=w190:bool)
        n93 = Compound Arithmetic op=AND(invert w205, w204, invert w203) -> (w199:bool)
        n94 = Compound Arithmetic op=AND(invert w200, w201, invert w202) -> (w198:bool)
        n95 = Compound Arithmetic op=AND(w199, w198) -> (w193:bool)
        n96 = Not(x=w193) -> (.not. x?=w187:bool)
        n97 = Compound Arithmetic op=AND(w193, w210, w211, invert w213, invert w214) -> (w207:bool)
        n98 = Compound Arithmetic op=AND(invert w191, invert w190, w187) -> (w192:bool)
        n99 = Select(t=w188, s=w187, f=w189) -> (s? t:f=w196:T11)
        n100 = Select(t=w188, s=w187, f=w189) -> (s? t:f=w197:T11)
        n101 = Select(t=w188, s=w192, f=w189) -> (s? t:f=w186:T11)
        n102 = Select(t=w188, s=w207, f=w189) -> (s? t:f=w208:T11)
        n103 = property on="Generate Root Certificate" class="Bool"("DisabledEnum"=w186) -> ()  [unwired: 2 in, 2 out]
        n104 = property on="Generate Server Certificates" class="Bool"("DisabledEnum"=w208) -> ()  [unwired: 2 in, 2 out]
        n105 = property on="Common Name" class="Str"("DisabledEnum"=w196) -> ()  [unwired: 2 in, 2 out]
        n106 = property on="hostname" class="Str"("DisabledEnum"=w197) -> ()  [unwired: 2 in, 2 out]
        n107 = call <vilib>:"Add State(s) to Queue__JKI_lib_State_Machine.vi"("State(s) in (\"\")"=w217) -> ("States Out"=w216:string)  [unwired: 14 in]
      }
      frame "UI: Display CA" {
        n108 = Unbundle By Name(w218) -> ()  [unwired: 1 out]
        n109 = call <vilib>:"Add State(s) to Queue__JKI_lib_State_Machine.vi"("State(s) in (\"\")"=w221) -> ("States Out"=w220:string)  [unwired: 14 in]
      }
      frame "UI: Display Server Cert" {
        n110 = Unbundle By Name(w222) -> ()  [unwired: 1 out]
        n111 = call <vilib>:"Add State(s) to Queue__JKI_lib_State_Machine.vi"("State(s) in (\"\")"=w225) -> ("States Out"=w224:string)  [unwired: 14 in]
      }
      frame "UI: Show Temporary Folder" {
        n112 = Unbundle By Name(w227) -> ("temp folder"=w226:path)
        n113 = call-poly <vilib>:"Open URL in Default Browser.vi"("path"=w226) -> ()  [unwired: 5 in, 2 out]
        n114 = call <vilib>:"Add State(s) to Queue__JKI_lib_State_Machine.vi"("State(s) in (\"\")"=w230) -> ("States Out"=w229:string)  [unwired: 14 in]
      }
      frame "UI: Cursor Set" {
        # "Argument"
        # "Set and Unset Cursor Busy.\n(Usage: \"UI: Cursor Set >> Busy|Idle\")"
        n115 = case shown="\"Idle\", Default" w231 {
          tunnel: w233 -> [w238 w240]
          tunnel: [w237 w239] -> w232
          frame "Idle", Default {
            n116 = call <vilib>:"Unset Busy.vi"("error in (no error)"=w238) -> ("error out"=w237:errorcluster)  [unwired: 10 in]
          }
          frame "Busy" {
            n117 = call <vilib>:"Set Busy.vi"("error in (no error)"=w240) -> ("error out"=w239:errorcluster)  [unwired: 9 in, 1 out]
          }
        }
        n118 = call <vilib>:"Add State(s) to Queue__JKI_lib_State_Machine.vi"("State(s) in (\"\")"=w236) -> ("States Out"=w235:string)  [unwired: 14 in]
      }
      frame "UI: Front Panel State" {
        # "Argument"
        # "Set Front Panel Open or Closed\n(Usage: \"UI: Front Panel State >> Open|Close\")"
        n119 = Unbundle By Name(w243) -> ("Core.Current VI Reference"=w242:refnum<vi>)
        n120 = case shown="\"Minimize\", \"Minimized\"" w241 {
          tunnel: w245 -> [w253 w268 w279 w292 w305]
          tunnel: [w255 w269 w281 w294 w307] -> w244
          tunnel: w242 -> [w254 w266 w280 w293 w306]
          frame "Open", "Standard", Default {
            w248 = T1."Standard" ("State")
            n121 = property class="VI"(reference=w254, error in=w253) -> (reference out=w251:refnum<vi>, error out=w252:errorcluster, "FP.State"=w250:T1)
            n122 = Not Equal?(x=w250, y=w248) -> (x != y?=w249:bool)
            n123 = case shown="True" w249 {
              tunnel: [w259 w261] -> w255
              tunnel: w252 -> [w258 w261]
              tunnel: w251 -> [w257 _]
              tunnel: w248 -> [w256 _]
              frame True {
                n124 = invoke class="VI" method="FP.Open"(reference=w257, error in=w258, "Activate"=TRUE, "State"=w256) -> (error out=w259:errorcluster)  [unwired: 1 in, 4 out]
              }
              frame False {
              }
            }
          }
          frame "Close", "Closed" {
            n125 = property class="VI"(reference=w266, error in=w268) -> (reference out=w265:refnum<vi>, error out=w267:errorcluster, "FP.State"=w263:T1)
            n126 = Not Equal?(x=w263, y=T1."Closed" ("Front Panel Window:State")) -> (x != y?=w262:bool)
            n127 = case shown="True" w262 {
              tunnel: [w270 w273] -> w269
              tunnel: w267 -> [w270 w272]
              tunnel: w265 -> [_ w271]
              frame False {
              }
              frame True {
                n128 = invoke class="VI" method="FP.Close"(reference=w271, error in=w272) -> (error out=w273:errorcluster)  [unwired: 1 in, 2 out]
              }
            }
          }
          frame "Hidden", "Hide" {
            w274 = T1."Hidden" ("State")
            n129 = property class="VI"(reference=w280, error in=w279) -> (reference out=w277:refnum<vi>, error out=w278:errorcluster, "FP.State"=w276:T1)
            n130 = Not Equal?(x=w276, y=w274) -> (x != y?=w275:bool)
            n131 = case shown="True" w275 {
              tunnel: [w285 w286] -> w281
              tunnel: w278 -> [w284 w286]
              tunnel: w277 -> [w283 _]
              tunnel: w274 -> [w282 _]
              frame True {
                n132 = invoke class="VI" method="FP.Open"(reference=w283, error in=w284, "State"=w282) -> (error out=w285:errorcluster)  [unwired: 2 in, 4 out]
              }
              frame False {
              }
            }
          }
          frame "Minimize", "Minimized" {
            w287 = T1."Minimized" ("State")
            n133 = property class="VI"(reference=w293, error in=w292) -> (reference out=w290:refnum<vi>, error out=w291:errorcluster, "FP.State"=w289:T1)
            n134 = Not Equal?(x=w289, y=w287) -> (x != y?=w288:bool)
            n135 = case shown="True" w288 {
              tunnel: [w298 w299] -> w294
              tunnel: w291 -> [w297 w299]
              tunnel: w290 -> [w296 _]
              tunnel: w287 -> [w295 _]
              frame True {
                n136 = invoke class="VI" method="FP.Open"(reference=w296, error in=w297, "State"=w295) -> (error out=w298:errorcluster)  [unwired: 2 in, 4 out]
              }
              frame False {
              }
            }
          }
          frame "Maximize", "Maximized" {
            w300 = T1."Maximized" ("State")
            n137 = property class="VI"(reference=w306, error in=w305) -> (reference out=w303:refnum<vi>, error out=w304:errorcluster, "FP.State"=w302:T1)
            n138 = Not Equal?(x=w302, y=w300) -> (x != y?=w301:bool)
            n139 = case shown="True" w301 {
              tunnel: [w311 w312] -> w307
              tunnel: w304 -> [w310 w312]
              tunnel: w303 -> [w309 _]
              tunnel: w300 -> [w308 _]
              frame True {
                n140 = invoke class="VI" method="FP.Open"(reference=w309, error in=w310, "State"=w308) -> (error out=w311:errorcluster)  [unwired: 2 in, 4 out]
              }
              frame False {
              }
            }
          }
        }
        n141 = call <vilib>:"Add State(s) to Queue__JKI_lib_State_Machine.vi"("State(s) in (\"\")"=w247) -> ("States Out"=w246:string)  [unwired: 14 in]
      }
      frame "---------- Macro ----------" {
        # "Do not put any code in this frame.\n(It is a separator no-op. You can make a copy of this frame to create a new Macro frame)"
        n142 = call <vilib>:"Add State(s) to Queue__JKI_lib_State_Machine.vi"("State(s) in (\"\")"=w316) -> ("States Out"=w315:string)  [unwired: 14 in]
      }
      frame "Macro: Initialize" {
        w317 = "Data: Initialize\nInitialize Core Data\nUI: Initialize\nUI: Front Panel State >> Open\n\nCFSSL: Find EXE\nCFSSL: Load Certification Authority\nCFSSL: Read CA Certificates\nCFSSL: Validate CA Certificates\nCFSSL: Create Temp Folder\nUI: List Certificates\nUI: Display Selected Certificate\nUI: Refresh"  # Data: Initialize Initialize Core Data UI: Initialize UI: Front Panel State >> Open  CFSSL: Find EXE CFSSL: Load Certification Authority CFSSL: Read CA Certificates CFSSL: Validate CA Certificates CFSSL: Create Temp Folder UI: List Certificates UI: Display Selected Certificate UI: Refresh
        # "Initialization Macro\n(This is called once, when the VI starts)"
        n143 = call <vilib>:"Add State(s) to Queue__JKI_lib_State_Machine.vi"("State(s) in Front (\"\")"=w317, "State(s) in (\"\")"=w321) -> ("States Out"=w320:string)  [unwired: 13 in]
      }
      frame "Macro: Generate Certification Authority" {
        n144 = call <vilib>:"Add State(s) to Queue__JKI_lib_State_Machine.vi"("State(s) in Front (\"\")"="CFSSL: Create Temp Folder\nCFSSL: Prepare CA Request File\nCFSSL: Generate Certification Authority\nCFSSL: Save CA Certificate\nCFSSL: Load Certification Authority\nCFSSL: Read CA Certificates\nCFSSL: Validate CA Certificates\nUI: Refresh\nUI: List Certificates\nUI: Display Selected Certificate", "State(s) in (\"\")"=w326) -> ("States Out"=w325:string)  [unwired: 13 in]
      }
      frame "Macro: Generate Server Certificate" {
        n145 = Bundle By Name(cluster=w330, "Processing Queue"="Servers") -> (w329:T9)
        n146 = call <vilib>:"Add State(s) to Queue__JKI_lib_State_Machine.vi"("State(s) in Front (\"\")"="CFSSL: Create Temp Folder\nCFSSL: Prepare Gencert Config File\nCFSSL: Copy Temporary CA Certificate\n\nMacro: Process Next Server", "State(s) in (\"\")"=w334, "State(s) at Back (\"\")"="UI: Refresh\nUI: List Certificates\nUI: Display Selected Certificate") -> ("States Out"=w333:string)  [unwired: 12 in]
      }
      frame "Macro: Export Root Bundle" {
        n147 = call <vilib>:"Add State(s) to Queue__JKI_lib_State_Machine.vi"("State(s) in Front (\"\")"="CFSSL: Export Root Certificate\nCFSSL: Export Root Private Key\nCFSSL: Export Root Signing Request", "State(s) in (\"\")"=w339) -> ("States Out"=w338:string)  [unwired: 13 in]
      }
      frame "Macro: Process Next Server" {
        n148 = Unbundle By Name(w345) -> ("Processing Queue"=w344:cluster{"hosts":string[], "name":string}[])
        n149 = Empty Array?(array=w344) -> (empty?=w343:bool)
        n150 = Select(t="UI: Refresh", s=w343, f="CFSSL: Load Next Server\nCFSSL: Prepare Server Request File\nCFSSL: Generate Server Certificate\nCFSSL: Save Temporary Server Certificate\nMacro: Process Next Server") -> (s? t:f=w340:string)
        n151 = call <vilib>:"Add State(s) to Queue__JKI_lib_State_Machine.vi"("State(s) in Front (\"\")"=w340, "State(s) in (\"\")"=w348) -> ("States Out"=w347:string)  [unwired: 13 in]
      }
      frame "Macro: Export Server Bundle" {
        n152 = call <vilib>:"Add State(s) to Queue__JKI_lib_State_Machine.vi"("State(s) in Front (\"\")"="CFSSL: Export Server Certificate\nCFSSL: Export Server Private Key\nCFSSL: Export Server Signing Request", "State(s) in (\"\")"=w353) -> ("States Out"=w352:string)  [unwired: 13 in]
      }
      frame "Macro: Exit" {
        # "Exit Macro\n(This is called once, when the VI exits)"
        n153 = Unbundle By Name(w361) -> ("Core.Close Panel on Exit?"=w360:bool)
        n154 = Select(t="UI: Front Panel State >> Close", s=w360, f="") -> (s? t:f=w357:string)
        n155 = call <vilib>:"Add State(s) to Queue__JKI_lib_State_Machine.vi"("State(s) in Front (\"\")"="CFSSL: Delete Temp Folder", "State(s) in (\"\")"=w357, "State(s) at Back (\"\")"="Data: Cleanup\nExit") -> ("States Out"=w355:string)  [unwired: 12 in]
        n156 = call <vilib>:"Add State(s) to Queue__JKI_lib_State_Machine.vi"("State(s) in Front (\"\")"=w355, "State(s) in (\"\")"=w364) -> ("States Out"=w363:string)  [unwired: 13 in]
      }
      frame "---------- Cloudflare SSL ----------" {
        n157 = call <vilib>:"Add State(s) to Queue__JKI_lib_State_Machine.vi"("State(s) in (\"\")"=w368) -> ("States Out"=w367:string)  [unwired: 14 in]
      }
      frame "CFSSL: Find EXE" {
        n158 = Current VI's Path() -> (path=w371:path)
        n159 = Build Path(base path=w371, name or relative path=path "../cfssl.exe") -> (appended path=w369:path)
        n160 = Bundle By Name(cluster=w373, "cfssl path"=w369) -> (w372:T9)
        n161 = call <vilib>:"Add State(s) to Queue__JKI_lib_State_Machine.vi"("State(s) in (\"\")"=w376) -> ("States Out"=w375:string)  [unwired: 14 in]
      }
      frame "CFSSL: Create Temp Folder" {
        n162 = call <userlib>:"Temporary Directory__ogtk.vi"("Relative path (.)"=path "LV_CFSSL") -> ("Temporary Directory (+ Relative)"=w380:path)
        n163 = call <userlib>:"Create Dir if Non-Existant__ogtk.vi"("error in (no error)"=w379, "Directory Path"=w380) -> ("error out"=w378:errorcluster, "dup Directory Path"=w377:path)  [unwired: 7 in, 1 out]
        n164 = Bundle By Name(cluster=w383, "temp folder"=w377) -> (w382:T9)
        n165 = call <vilib>:"Add State(s) to Queue__JKI_lib_State_Machine.vi"("State(s) in (\"\")"=w385) -> ("States Out"=w384:string)  [unwired: 14 in]
      }
      frame "CFSSL: Delete Temp Folder" {
        n166 = Unbundle By Name(w393) -> ("temp folder"=w387:path)
        n167 = Empty String/Path?(string/path=w387) -> (empty?=w386:bool)
        n168 = call-poly <userlib>:"File Exists__ogtk.vi"("file path"=w387) -> ("is directory"=w391:bool, "exists"=w392:bool)  [unwired: 6 in]
        n169 = Compound Arithmetic op=AND(w391, w392, invert w386) -> (w390:bool)
        n170 = case shown="True" w390 {
          tunnel: w387 -> [_ w400]
          tunnel: [w396 w398] -> w389
          tunnel: w388 -> [w396 w399]
          frame False {
          }
          frame True {
            w397 = TRUE ("Recursive? (FALSE)")
            n171 = call <userlib>:"Delete Recursive__ogtk.vi"("error in (no error)"=w399, "Ignore Read-Only? (FALSE)"=w397, "Recursive? (FALSE)"=w397, "Path"=w400) -> ("error out"=w398:errorcluster)  [unwired: 6 in, 1 out]
          }
        }
        n172 = call <vilib>:"Add State(s) to Queue__JKI_lib_State_Machine.vi"("State(s) in (\"\")"=w395) -> ("States Out"=w394:string)  [unwired: 14 in]
      }
      frame "CFSSL: Load Certification Authority" {
        n173 = Unbundle By Name(w418) -> ("Certificates Folder"=w402:path)
        n174 = Build Path(base path=w402, name or relative path="root.crt") -> (appended path=w403:path)
        n175 = Build Path(base path=w402, name or relative path="root-key.pem") -> (appended path=w401:path)
        n176 = call-poly <userlib>:"File Exists__ogtk.vi"("file path"=w403) -> ("is directory"=w416:bool, "exists"=w415:bool)  [unwired: 6 in]
        n177 = Empty String/Path?(string/path=w403) -> (empty?=w414:bool)
        n178 = call-poly <userlib>:"File Exists__ogtk.vi"("file path"=w401) -> ("is directory"=w406:bool, "exists"=w407:bool)  [unwired: 6 in]
        n179 = Empty String/Path?(string/path=w401) -> (empty?=w408:bool)
        n180 = Compound Arithmetic op=AND(invert w416, w415, invert w414) -> (w413:bool)
        n181 = Compound Arithmetic op=AND(invert w406, w407, invert w408) -> (w409:bool)
        n182 = Select(t=w403, s=w413, f=path "") -> (s? t:f=w411:path)
        n183 = Select(t=w401, s=w409, f=path "") -> (s? t:f=w404:path)
        n184 = Bundle By Name(cluster=w418, "Root Certificate"=w411, "Root Private Key"=w404) -> (w419:T9)
        n185 = call <vilib>:"Add State(s) to Queue__JKI_lib_State_Machine.vi"("State(s) in (\"\")"=w422) -> ("States Out"=w421:string)  [unwired: 14 in]
      }
      frame "CFSSL: Generate Certification Authority" {
        n186 = Unbundle By Name(w426) -> ("cfssl path"=w432:path, "temp folder"=w431:path)
        n187 = Format Into String(format string="%s gencert -initca csr-ca.json", w432) -> (resulting string=w434:string)  [unwired: 2 in, 1 out]
        n188 = call <vilib>:"System Exec.vi"("run minimized? (F)"=TRUE, "error in (no error)"=w424, "working directory"=w431, "command line"=w434) -> ("error out"=w429:errorcluster, "standard output"=w430:string)  [unwired: 4 in, 2 out]
        n189 = Unbundle By Name(w426) -> ("CA"=w425:T8)
        n190 = Unflatten From JSON(JSON string=w430, type and defaults=w425, error in (no error)=w429) -> (value=w428:T8, error out=w423:errorcluster)  [unwired: 4 in]
        n191 = Bundle By Name(cluster=w426, "CA"=w428) -> (w427:T9)
        n192 = call <vilib>:"Add State(s) to Queue__JKI_lib_State_Machine.vi"("State(s) in (\"\")"=w437) -> ("States Out"=w436:string)  [unwired: 14 in]
      }
      frame "CFSSL: Generate Server Certificate" {
        n193 = Unbundle By Name(w442) -> ("cfssl path"=w448:path, "temp folder"=w447:path)
        n194 = Format Into String(format string="\"%s\" gencert -ca ca.pem -ca-key ca-key.pem -config config.json csr-server.json" ("command line"), w448) -> (resulting string=w449:string)  [unwired: 2 in, 1 out]
        n195 = call <vilib>:"System Exec.vi"("run minimized? (F)"=TRUE, "error in (no error)"=w440, "working directory"=w447, "command line"=w449) -> ("error out"=w445:errorcluster, "standard output"=w446:string)  [unwired: 4 in, 2 out]
        n196 = Unbundle By Name(w442) -> ("Server"=w441:T8)
        n197 = Unflatten From JSON(JSON string=w446, type and defaults=w441, error in (no error)=w445) -> (value=w444:T8, error out=w439:errorcluster)  [unwired: 4 in]
        n198 = Bundle By Name(cluster=w442, "Server"=w444) -> (w443:T9)
        n199 = call <vilib>:"Add State(s) to Queue__JKI_lib_State_Machine.vi"("State(s) in (\"\")"=w452) -> ("States Out"=w451:string)  [unwired: 14 in]
      }
      frame "CFSSL: Prepare CA Request File" {
        (unwired) "{\n    \"CN\": \"lvtls-ca.example\",\n    \"hosts\": [\"lvtls-ca.example\"],\n    \"key\": {\"algo\": \"ecdsa\", \"size\": 256},\n    \"names\": [],\n    \"ca\": {\"pathlen\": 1, \"expiry\": \"143800h\"}\n}" ("name or relative path")
        # "https://github.com/cloudflare/cfssl/wiki/Creating-a-new-CSR"
        n200 = Unbundle By Name(w473) -> ("temp folder"=w472:path)
        n201 = call-poly <userlib>:"Build Path__ogtk.vi"("name or relative path"="csr-ca.json", "base path"=w472) -> ("appended path"=w461:path)
        n202 = Bundle By Name(cluster=T4 {"CN"="", "hosts"=[], "key"={"algo"="ecdsa", "size"=256}, "ca"={"pathlen"=0, "expiry"=""}} ("CSR"), "CN"="Common Name", "hosts"="Hosts", "key.algo"="ecdsa", "key.size"=u32 256, "ca.pathlen"=u8 1, "ca.expiry"="143800h") -> (w467:T4)
        n203 = Flatten To JSON(anything=w467, error in (no error)=w454) -> (JSON string=w459:string, 11:w455:errorcluster)  [unwired: 1 in]
        n204 = Open/Create/Replace File(file path (use dialog)=w461, error in=w455, operation (0:open)=T3."replace or create") -> (refnum out=w460:refnum<file>, error out=w462:errorcluster)  [unwired: 3 in, 1 out]
        n205 = Write to Text File(file (use dialog)=w460, text=w459, error in=w462) -> (refnum out=w456:refnum<file>, error out=w457:errorcluster)  [unwired: 1 in, 1 out]
        n206 = Close File(refnum=w456, error in=w457) -> (error out=w453:errorcluster)  [unwired: 1 out]
        n207 = call <vilib>:"Add State(s) to Queue__JKI_lib_State_Machine.vi"("State(s) in (\"\")"=w475) -> ("States Out"=w474:string)  [unwired: 14 in]
      }
      frame "CFSSL: Prepare Server Request File" {
        (unwired) "{\n    \"CN\": \"lvtls.example\",\n    \"hosts\": [\"lvtls.example\"],\n    \"key\": {\"algo\": \"ecdsa\", \"size\": 256},\n    \"names\": []\n}" ("name or relative path")
        # "https://github.com/cloudflare/cfssl/wiki/Creating-a-new-CSR"
        n208 = Unbundle By Name(w494) -> ("temp folder"=w493:path, "Active CN"=w477:string, "Active Hosts"=w476:string[])
        n209 = call-poly <userlib>:"Build Path__ogtk.vi"("name or relative path"="csr-server.json", "base path"=w493) -> ("appended path"=w490:path)
        n210 = Bundle By Name(cluster=T7 {"CN"="", "hosts"=[], "key"={"algo"="ecdsa", "size"=256}} ("CSR"), "CN"=w477, "hosts"=w476, "key.algo"="ecdsa", "key.size"=u32 256) -> (w479:T7)
        n211 = Flatten To JSON(anything=w479, error in (no error)=w483) -> (JSON string=w488:string, 11:w484:errorcluster)  [unwired: 1 in]
        n212 = Open/Create/Replace File(file path (use dialog)=w490, error in=w484, operation (0:open)=T3."replace or create") -> (refnum out=w489:refnum<file>, error out=w491:errorcluster)  [unwired: 3 in, 1 out]
        n213 = Write to Text File(file (use dialog)=w489, text=w488, error in=w491) -> (refnum out=w485:refnum<file>, error out=w486:errorcluster)  [unwired: 1 in, 1 out]
        n214 = Close File(refnum=w485, error in=w486) -> (error out=w482:errorcluster)  [unwired: 1 out]
        n215 = call <vilib>:"Add State(s) to Queue__JKI_lib_State_Machine.vi"("State(s) in (\"\")"=w496) -> ("States Out"=w495:string)  [unwired: 14 in]
      }
      frame "CFSSL: Copy Temporary CA Certificate" {
        n216 = Unbundle By Name(w506) -> ("Root Certificate"=w510:path, "temp folder"=w511:path)
        n217 = Unbundle By Name(w506) -> ("Root Private Key"=w503:path, "temp folder"=w501:path)
        n218 = call-poly <userlib>:"Build Path__ogtk.vi"("name or relative path"="ca-key.pem", "base path"=w501) -> ("appended path"=w504:path)
        n219 = call-poly <userlib>:"Build Path__ogtk.vi"("name or relative path"="ca.pem", "base path"=w511) -> ("appended path"=w508:path)
        n220 = call <userlib>:"Copy with Options__ogtk.vi"("error in (no error)"=w500, "Replace Mode (Never)"=enum16{"Never", "Always", "If Newer"}."Always", "target path"=w504, "source path"=w503) -> ("error out"=w497:errorcluster)  [unwired: 6 in, 1 out]
        n221 = call <userlib>:"Copy with Options__ogtk.vi"("error in (no error)"=w500, "Replace Mode (Never)"=enum16{"Never", "Always", "If Newer"}."Always", "target path"=w508, "source path"=w510) -> ("error out"=w498:errorcluster)  [unwired: 6 in, 1 out]
        n222 = Merge Errors(w498, w497) -> (w499:errorcluster)
        n223 = call <vilib>:"Add State(s) to Queue__JKI_lib_State_Machine.vi"("State(s) in (\"\")"=w513) -> ("States Out"=w512:string)  [unwired: 14 in]
      }
      frame "CFSSL: Load Next Server" {
        n224 = Unbundle By Name(w518) -> ("Processing Queue"=w517:cluster{"hosts":string[], "name":string}[])
        n225 = Delete From Array(array=w517) -> (deleted portion=w515:cluster{"hosts":string[], "name":string}, array with subset deleted=w516:cluster{"hosts":string[], "name":string}[])  [unwired: 2 in]
        n226 = Unbundle By Name(w515) -> ("name"=w520:string, "hosts"=w519:string[])
        n227 = Bundle By Name(cluster=w518, "Processing Queue"=w516, "Active CN"=w520, "Active Hosts"=w519) -> (w521:T9)
        n228 = call <vilib>:"Add State(s) to Queue__JKI_lib_State_Machine.vi"("State(s) in (\"\")"=w523) -> ("States Out"=w522:string)  [unwired: 14 in]
      }
      frame "CFSSL: Prepare Gencert Config File" {
        n229 = Unbundle By Name(w535) -> ("temp folder"=w534:path)
        n230 = call-poly <userlib>:"Build Path__ogtk.vi"("name or relative path"="config.json", "base path"=w534) -> ("appended path"=w531:path)
        n231 = Open/Create/Replace File(file path (use dialog)=w531, error in=w524, operation (0:open)=T3."replace or create") -> (refnum out=w530:refnum<file>, error out=w532:errorcluster)  [unwired: 3 in, 1 out]
        n232 = Write to Text File(file (use dialog)=w530, text="{\n  \"signing\": {\n       \"default\": {\n           \"expiry\": \"143800h\", \n           \"usages\": [\"server auth\"]\n        }\n    }\n}" ("name or relative path"), error in=w532) -> (refnum out=w527:refnum<file>, error out=w528:errorcluster)  [unwired: 1 in, 1 out]
        n233 = Close File(refnum=w527, error in=w528) -> (error out=w526:errorcluster)  [unwired: 1 out]
        n234 = call <vilib>:"Add State(s) to Queue__JKI_lib_State_Machine.vi"("State(s) in (\"\")"=w537) -> ("States Out"=w536:string)  [unwired: 14 in]
      }
      frame "CFSSL: Save CA Certificate" {
        w546 = T3."replace or create with confirmation" ("operation (0:open)")
        n235 = Unbundle By Name(w538) -> ("Certificates Folder"=w559:path)
        n236 = Unbundle By Name(w538) -> ("CA.cert"=w558:string)
        n237 = Unbundle By Name(w538) -> ("CA.key"=w547:string)
        n238 = Unbundle By Name(w538) -> ("CA.csr"=w548:string)
        n239 = call-poly <userlib>:"Build Path__ogtk.vi"("name or relative path"="root.csr", "base path"=w559) -> ("appended path"=w553:path)
        n240 = call-poly <userlib>:"Build Path__ogtk.vi"("name or relative path"="root.crt", "base path"=w559) -> ("appended path"=w540:path)
        n241 = call-poly <userlib>:"Build Path__ogtk.vi"("name or relative path"="root-key.pem", "base path"=w559) -> ("appended path"=w539:path)
        n242 = Open/Create/Replace File(file path (use dialog)=w553, operation (0:open)=w546) -> (refnum out=w555:refnum<file>, error out=w554:errorcluster)  [unwired: 4 in, 1 out]
        n243 = Open/Create/Replace File(file path (use dialog)=w539, operation (0:open)=w546) -> (refnum out=w551:refnum<file>, error out=w552:errorcluster)  [unwired: 4 in, 1 out]
        n244 = Open/Create/Replace File(file path (use dialog)=w540, operation (0:open)=w546) -> (refnum out=w564:refnum<file>, error out=w565:errorcluster)  [unwired: 4 in, 1 out]
        n245 = Write to Text File(file (use dialog)=w555, text=w548, error in=w554) -> (refnum out=w557:refnum<file>, error out=w556:errorcluster)  [unwired: 1 in, 1 out]
        n246 = Write to Text File(file (use dialog)=w551, text=w547, error in=w552) -> (refnum out=w549:refnum<file>, error out=w550:errorcluster)  [unwired: 1 in, 1 out]
        n247 = Write to Text File(file (use dialog)=w564, text=w558, error in=w565) -> (refnum out=w562:refnum<file>, error out=w563:errorcluster)  [unwired: 1 in, 1 out]
        n248 = Close File(refnum=w557, error in=w556) -> (error out=w543:errorcluster)  [unwired: 1 out]
        n249 = Close File(refnum=w549, error in=w550) -> (error out=w542:errorcluster)  [unwired: 1 out]
        n250 = Close File(refnum=w562, error in=w563) -> (error out=w544:errorcluster)  [unwired: 1 out]
        n251 = Merge Errors(w545, w544, w543, w542) -> (w541:errorcluster)
        n252 = call <vilib>:"Add State(s) to Queue__JKI_lib_State_Machine.vi"("State(s) in (\"\")"=w568) -> ("States Out"=w567:string)  [unwired: 14 in]
      }
      frame "CFSSL: Read CA Certificates" {
        n253 = Unbundle By Name(w584) -> ("Certificates Folder"=w585:path)
        n254 = call-poly <userlib>:"Build Path__ogtk.vi"("name or relative path"="root-key.pem", "base path"=w585) -> ("appended path"=w570:path)
        n255 = call-poly <userlib>:"Build Path__ogtk.vi"("name or relative path"="root.crt", "base path"=w585) -> ("appended path"=w575:path)
        n256 = call-poly <userlib>:"File Exists__ogtk.vi"("file path"=w575) -> ("is directory"=w578:bool, "exists"=w577:bool)  [unwired: 6 in]
        n257 = Empty String/Path?(string/path=w575) -> (empty?=w576:bool)
        n258 = call-poly <userlib>:"File Exists__ogtk.vi"("file path"=w570) -> ("is directory"=w571:bool, "exists"=w572:bool)  [unwired: 6 in]
        n259 = Empty String/Path?(string/path=w570) -> (empty?=w573:bool)
        n260 = Compound Arithmetic op=AND(invert w578, w577, invert w576) -> (w574:bool)
        n261 = Compound Arithmetic op=AND(invert w571, w572, invert w573) -> (w569:bool)
        n262 = case shown="True" w574 {
          tunnel: w575 -> [_ w608]
          tunnel: [_ w604] -> w582
          tunnel: [_ w601] -> w581
          frame False {
          }
          frame True {
            n263 = Open/Create/Replace File(file path (use dialog)=w608, operation (0:open)=T3."open", access (0:read/write)=enum16{"read/write", "read-only", "write-only"}."read-only") -> (refnum out=w607:refnum<file>, error out=w609:errorcluster)  [unwired: 3 in, 1 out]
            n264 = Read from Text File(file (use dialog)=w607, error in=w609) -> (refnum out=w605:refnum<file>, text=w604:string, error out=w606:errorcluster)  [unwired: 2 in, 1 out]
            n265 = Close File(refnum=w605, error in=w606) -> (error out=w601:errorcluster)  [unwired: 1 out]
          }
        }
        n266 = case shown="True" w569 {
          tunnel: w570 -> [_ w596]
          tunnel: [_ w595] -> w580
          tunnel: [_ w592] -> w579
          frame False {
          }
          frame True {
            n267 = Open/Create/Replace File(file path (use dialog)=w596, operation (0:open)=T3."open", access (0:read/write)=enum16{"read/write", "read-only", "write-only"}."read-only") -> (refnum out=w598:refnum<file>, error out=w597:errorcluster)  [unwired: 3 in, 1 out]
            n268 = Read from Text File(file (use dialog)=w598, error in=w597) -> (refnum out=w600:refnum<file>, text=w592:string, error out=w599:errorcluster)  [unwired: 2 in, 1 out]
            n269 = Close File(refnum=w600, error in=w599) -> (error out=w595:errorcluster)  [unwired: 1 out]
          }
        }
        n270 = Bundle By Name(cluster=w584, "CA.cert"=w582, "CA.key"=w579) -> (w583:T9)
        n271 = Merge Errors(w587, w581, w580) -> (w586:errorcluster)
        n272 = call <vilib>:"Add State(s) to Queue__JKI_lib_State_Machine.vi"("State(s) in (\"\")"=w591) -> ("States Out"=w590:string)  [unwired: 14 in]
      }
      frame "CFSSL: Validate CA Certificates" {
        n273 = Unbundle By Name(w613) -> ("Root Certificate"=w611:path, "Root Private Key"=w610:path)  [unwired: 2 out]
        n274 = Bundle By Name(cluster=w613, "Root Certificate"=w611, "Root Private Key"=w610) -> (w612:T9)
        n275 = Merge Errors(w615) -> (w614:errorcluster)
        n276 = call <vilib>:"Add State(s) to Queue__JKI_lib_State_Machine.vi"("State(s) in (\"\")"=w617) -> ("States Out"=w616:string)  [unwired: 14 in]
      }
      frame "CFSSL: Save Temporary CA Certificate" {
        w618 = T3."replace or create with confirmation" ("operation (0:open)")
        n277 = Unbundle By Name(w630) -> ("temp folder"=w631:path)
        n278 = Unbundle By Name(w630) -> ("CA.cert"=w629:string)
        n279 = Unbundle By Name(w630) -> ("CA.key"=w623:string)
        n280 = call-poly <userlib>:"Build Path__ogtk.vi"("name or relative path"="root.crt", "base path"=w631) -> ("appended path"=w636:path)
        n281 = call-poly <userlib>:"Build Path__ogtk.vi"("name or relative path"="root-key.pem", "base path"=w631) -> ("appended path"=w624:path)
        n282 = Open/Create/Replace File(file path (use dialog)=w624, operation (0:open)=w618) -> (refnum out=w627:refnum<file>, error out=w628:errorcluster)  [unwired: 4 in, 1 out]
        n283 = Open/Create/Replace File(file path (use dialog)=w636, operation (0:open)=w618) -> (refnum out=w635:refnum<file>, error out=w637:errorcluster)  [unwired: 4 in, 1 out]
        n284 = Write to Text File(file (use dialog)=w627, text=w623, error in=w628) -> (refnum out=w625:refnum<file>, error out=w626:errorcluster)  [unwired: 1 in, 1 out]
        n285 = Write to Text File(file (use dialog)=w635, text=w629, error in=w637) -> (refnum out=w633:refnum<file>, error out=w634:errorcluster)  [unwired: 1 in, 1 out]
        n286 = Close File(refnum=w625, error in=w626) -> (error out=w620:errorcluster)  [unwired: 1 out]
        n287 = Close File(refnum=w633, error in=w634) -> (error out=w621:errorcluster)  [unwired: 1 out]
        n288 = Merge Errors(w622, w621, w620) -> (w619:errorcluster)
        n289 = call <vilib>:"Add State(s) to Queue__JKI_lib_State_Machine.vi"("State(s) in (\"\")"=w640) -> ("States Out"=w639:string)  [unwired: 14 in]
      }
      frame "CFSSL: Save Temporary Server Certificate" {
        w660 = T3."replace or create" ("operation (0:open)")
        n290 = Unbundle By Name(w655) -> ("Certificates Folder"=w651:path, "Active CN"=w647:string)
        n291 = Unbundle By Name(w655) -> ("Certificates Folder"=w650:path, "Active CN"=w654:string, "Server.key"=w649:string)
        n292 = Unbundle By Name(w655) -> ("Server.cert"=w641:string, "CA.cert"=w643:string)
        n293 = Format Into String(format string="%s-key.pem", w654) -> (resulting string=w652:string)  [unwired: 2 in, 1 out]
        n294 = Format Into String(format string="%s.crt", w647) -> (resulting string=w648:string)  [unwired: 2 in, 1 out]
        n295 = call-poly <userlib>:"Build Path__ogtk.vi"("name or relative path"=w648, "base path"=w651) -> ("appended path"=w669:path)
        n296 = call-poly <userlib>:"Build Path__ogtk.vi"("name or relative path"=w652, "base path"=w650) -> ("appended path"=w661:path)
        n297 = Open/Create/Replace File(file path (use dialog)=w661, operation (0:open)=w660) -> (refnum out=w664:refnum<file>, error out=w665:errorcluster)  [unwired: 4 in, 1 out]
        n298 = Open/Create/Replace File(file path (use dialog)=w669, operation (0:open)=w660) -> (refnum out=w668:refnum<file>, error out=w670:errorcluster)  [unwired: 4 in, 1 out]
        n299 = Write to Text File(file (use dialog)=w664, text=w649, error in=w665) -> (refnum out=w662:refnum<file>, error out=w663:errorcluster)  [unwired: 1 in, 1 out]
        n300 = Format Into String(format string="%s%s%s", w641, "\n", w643) -> (resulting string=w642:string)  [unwired: 2 in, 1 out]
        n301 = Close File(refnum=w662, error in=w663) -> (error out=w657:errorcluster)  [unwired: 1 out]
        n302 = Write to Text File(file (use dialog)=w668, text=w642, error in=w670) -> (refnum out=w666:refnum<file>, error out=w667:errorcluster)  [unwired: 1 in, 1 out]
        n303 = Close File(refnum=w666, error in=w667) -> (error out=w658:errorcluster)  [unwired: 1 out]
        n304 = Merge Errors(w659, w658, w657) -> (w656:errorcluster)
        n305 = call <vilib>:"Add State(s) to Queue__JKI_lib_State_Machine.vi"("State(s) in (\"\")"=w672) -> ("States Out"=w671:string)  [unwired: 14 in]
      }
      frame "CFSSL: Export Root Private Key" {
        n306 = Unbundle By Name(w681) -> ("Certificates Folder"=w682:path, "Root name"=w675:string)
        n307 = Unbundle By Name(w681) -> ("CA.key"=w680:string)
        n308 = call-poly <userlib>:"Convert File Extension__ogtk.vi"("new ending (none)"="pem" ("format string"), "file name"=w675) -> ("new filename"=w673:string)  [unwired: 1 out]
        n309 = call-poly <userlib>:"Build Path__ogtk.vi"("name or relative path"=w673, "base path"=w682) -> ("appended path"=w686:path)
        n310 = Open/Create/Replace File(file path (use dialog)=w686, operation (0:open)=T3."replace or create with confirmation") -> (refnum out=w685:refnum<file>, error out=w687:errorcluster)  [unwired: 4 in, 1 out]
        n311 = Write to Text File(file (use dialog)=w685, text=w680, error in=w687) -> (refnum out=w683:refnum<file>, error out=w684:errorcluster)  [unwired: 1 in, 1 out]
        n312 = Close File(refnum=w683, error in=w684) -> (error out=w677:errorcluster)  [unwired: 1 out]
        n313 = Merge Errors(w678, w677) -> (w676:errorcluster)
        n314 = call <vilib>:"Add State(s) to Queue__JKI_lib_State_Machine.vi"("State(s) in (\"\")"=w689) -> ("States Out"=w688:string)  [unwired: 14 in]
      }
      frame "CFSSL: Export Root Certificate" {
        n315 = Unbundle By Name(w698) -> ("Certificates Folder"=w699:path, "Root name"=w692:string)
        n316 = Unbundle By Name(w698) -> ("CA.cert"=w697:string)
        n317 = call-poly <userlib>:"Convert File Extension__ogtk.vi"("new ending (none)"="crt" ("format string"), "file name"=w692) -> ("new filename"=w690:string)  [unwired: 1 out]
        n318 = call-poly <userlib>:"Build Path__ogtk.vi"("name or relative path"=w690, "base path"=w699) -> ("appended path"=w703:path)
        n319 = Open/Create/Replace File(file path (use dialog)=w703, operation (0:open)=T3."replace or create with confirmation") -> (refnum out=w702:refnum<file>, error out=w704:errorcluster)  [unwired: 4 in, 1 out]
        n320 = Write to Text File(file (use dialog)=w702, text=w697, error in=w704) -> (refnum out=w700:refnum<file>, error out=w701:errorcluster)  [unwired: 1 in, 1 out]
        n321 = Close File(refnum=w700, error in=w701) -> (error out=w694:errorcluster)  [unwired: 1 out]
        n322 = Merge Errors(w695, w694) -> (w693:errorcluster)
        n323 = call <vilib>:"Add State(s) to Queue__JKI_lib_State_Machine.vi"("State(s) in (\"\")"=w706) -> ("States Out"=w705:string)  [unwired: 14 in]
      }
      frame "CFSSL: Export Root Signing Request" {
        n324 = Unbundle By Name(w715) -> ("Certificates Folder"=w716:path, "Root name"=w709:string)
        n325 = Unbundle By Name(w715) -> ("CA.csr"=w714:string)
        n326 = call-poly <userlib>:"Convert File Extension__ogtk.vi"("new ending (none)"="csr" ("format string"), "file name"=w709) -> ("new filename"=w707:string)  [unwired: 1 out]
        n327 = call-poly <userlib>:"Build Path__ogtk.vi"("name or relative path"=w707, "base path"=w716) -> ("appended path"=w720:path)
        n328 = Open/Create/Replace File(file path (use dialog)=w720, operation (0:open)=T3."replace or create with confirmation") -> (refnum out=w719:refnum<file>, error out=w721:errorcluster)  [unwired: 4 in, 1 out]
        n329 = Write to Text File(file (use dialog)=w719, text=w714, error in=w721) -> (refnum out=w717:refnum<file>, error out=w718:errorcluster)  [unwired: 1 in, 1 out]
        n330 = Close File(refnum=w717, error in=w718) -> (error out=w711:errorcluster)  [unwired: 1 out]
        n331 = Merge Errors(w712, w711) -> (w710:errorcluster)
        n332 = call <vilib>:"Add State(s) to Queue__JKI_lib_State_Machine.vi"("State(s) in (\"\")"=w723) -> ("States Out"=w722:string)  [unwired: 14 in]
      }
      frame "CFSSL: Export Server Certificate" {
        n333 = Unbundle By Name(w732) -> ("Certificates Folder"=w733:path, "Root name"=w726:string)
        n334 = Unbundle By Name(w732) -> ("Server.cert"=w731:string)
        n335 = call-poly <userlib>:"Convert File Extension__ogtk.vi"("new ending (none)"="cer" ("format string"), "file name"=w726) -> ("new filename"=w724:string)  [unwired: 1 out]
        n336 = call-poly <userlib>:"Build Path__ogtk.vi"("name or relative path"=w724, "base path"=w733) -> ("appended path"=w737:path)
        n337 = Open/Create/Replace File(file path (use dialog)=w737, operation (0:open)=T3."replace or create with confirmation") -> (refnum out=w736:refnum<file>, error out=w738:errorcluster)  [unwired: 4 in, 1 out]
        n338 = Write to Text File(file (use dialog)=w736, text=w731, error in=w738) -> (refnum out=w734:refnum<file>, error out=w735:errorcluster)  [unwired: 1 in, 1 out]
        n339 = Close File(refnum=w734, error in=w735) -> (error out=w728:errorcluster)  [unwired: 1 out]
        n340 = Merge Errors(w729, w728) -> (w727:errorcluster)
        n341 = call <vilib>:"Add State(s) to Queue__JKI_lib_State_Machine.vi"("State(s) in (\"\")"=w740) -> ("States Out"=w739:string)  [unwired: 14 in]
      }
      frame "CFSSL: Export Server Private Key" {
        n342 = Unbundle By Name(w749) -> ("Certificates Folder"=w750:path, "Root name"=w743:string)
        n343 = Unbundle By Name(w749) -> ("Server.key"=w748:string)
        n344 = call-poly <userlib>:"Convert File Extension__ogtk.vi"("new ending (none)"="pem" ("format string"), "file name"=w743) -> ("new filename"=w741:string)  [unwired: 1 out]
        n345 = call-poly <userlib>:"Build Path__ogtk.vi"("name or relative path"=w741, "base path"=w750) -> ("appended path"=w754:path)
        n346 = Open/Create/Replace File(file path (use dialog)=w754, operation (0:open)=T3."replace or create with confirmation") -> (refnum out=w753:refnum<file>, error out=w755:errorcluster)  [unwired: 4 in, 1 out]
        n347 = Write to Text File(file (use dialog)=w753, text=w748, error in=w755) -> (refnum out=w751:refnum<file>, error out=w752:errorcluster)  [unwired: 1 in, 1 out]
        n348 = Close File(refnum=w751, error in=w752) -> (error out=w745:errorcluster)  [unwired: 1 out]
        n349 = Merge Errors(w746, w745) -> (w744:errorcluster)
        n350 = call <vilib>:"Add State(s) to Queue__JKI_lib_State_Machine.vi"("State(s) in (\"\")"=w757) -> ("States Out"=w756:string)  [unwired: 14 in]
      }
      frame "CFSSL: Export Server Signing Request" {
        n351 = Unbundle By Name(w766) -> ("Certificates Folder"=w767:path, "Root name"=w760:string)
        n352 = Unbundle By Name(w766) -> ("Server.csr"=w765:string)
        n353 = call-poly <userlib>:"Convert File Extension__ogtk.vi"("new ending (none)"="csr" ("format string"), "file name"=w760) -> ("new filename"=w758:string)  [unwired: 1 out]
        n354 = call-poly <userlib>:"Build Path__ogtk.vi"("name or relative path"=w758, "base path"=w767) -> ("appended path"=w771:path)
        n355 = Open/Create/Replace File(file path (use dialog)=w771, operation (0:open)=T3."replace or create with confirmation") -> (refnum out=w770:refnum<file>, error out=w772:errorcluster)  [unwired: 4 in, 1 out]
        n356 = Write to Text File(file (use dialog)=w770, text=w765, error in=w772) -> (refnum out=w768:refnum<file>, error out=w769:errorcluster)  [unwired: 1 in, 1 out]
        n357 = Close File(refnum=w768, error in=w769) -> (error out=w762:errorcluster)  [unwired: 1 out]
        n358 = Merge Errors(w763, w762) -> (w761:errorcluster)
        n359 = call <vilib>:"Add State(s) to Queue__JKI_lib_State_Machine.vi"("State(s) in (\"\")"=w774) -> ("States Out"=w773:string)  [unwired: 14 in]
      }
    }
  }
